vi "Ref AVI Video-Generate file name.vi"(8 "error in (no error)":errorcluster, 9 "Channel":T1, 11 "Videos folder path":path) -> (0 "error out":errorcluster, 3 "AVI file path & name":path)   [LabVIEW 2020]
uses:
  Typedefs/Channel Selector.ctl
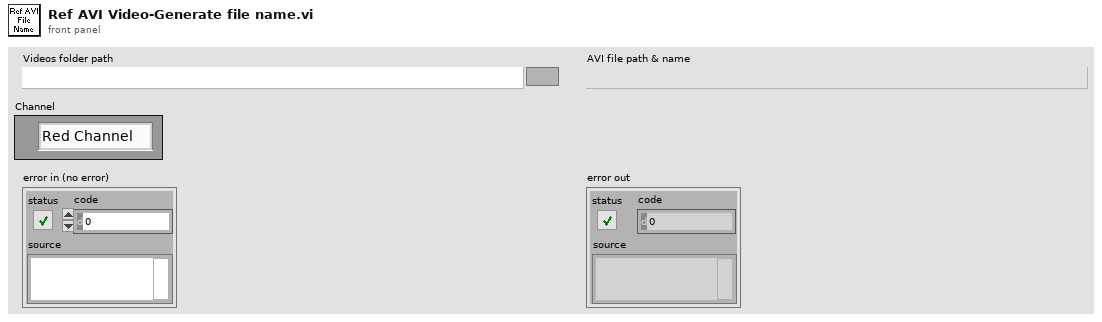
[diagram p1: front panel]
types:
  T1 = typedef "Channel Selector.ctl" = enum16{"Red Channel", "Green Channel", "Blended"}
  T2 = typedef "AVI Refs cluster.ctl" = cluster{"AVI2 path":path, "AVI 2 Refnum":T3, "New Image":T4, "error out":errorcluster, "Avi 1 Refnum":T5}
  T3 = typedef "IMAQ AVI2 Refnum.ctl" = refnum<k20>
  T4 = typedef "IMAQ Image.ctl" = refnum<image>
  T5 = typedef "AviRefnum.ctl" = refnum<k1>
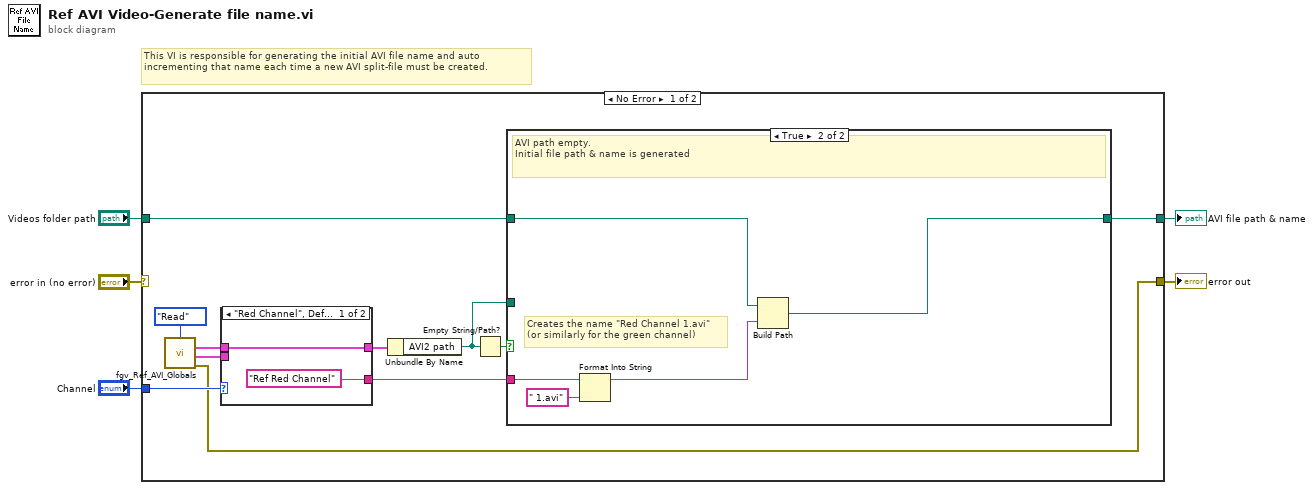
[diagram p0: block diagram]
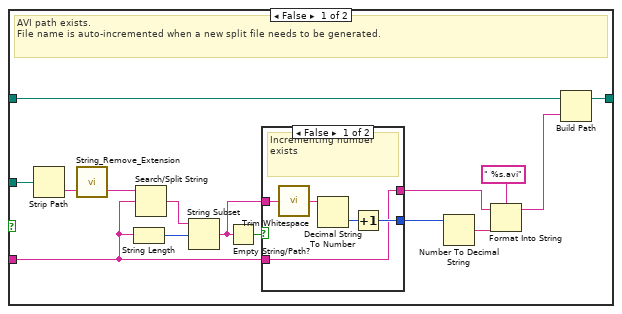
[diagram p2: hidden frame]
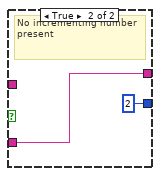
[diagram p3: hidden frame]
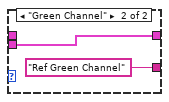
[diagram p4: hidden frame]
diagram:
  # "This VI is responsible for generating the initial AVI file name and auto incrementing that name each time a new AVI split-file must be created."
  n1 = case shown="No Error" "error in (no error)" {
    selector: "error in (no error)" -> [_ w49]
    tunnel: "Videos folder path" -> [w11 w48]
    tunnel: [w9 w48] -> w4
    tunnel: [w7 w49] -> w3
    tunnel: "Channel" -> [w8 _]
    frame No Error {
      n2 = call "fgv_Ref_AVI_Globals.vi"("Function"=enum16{"Intialize", "Write", "Read", "Clear"}."Read") -> ("Red Ref AVI"=w14:T2, "Green Ref AVI"=w15:T2, "error out"=w7:errorcluster)  [unwired: 11 in, 1 out]
      n3 = case shown="\"Red Channel\", Default" w8 {
        tunnel: w14 -> [w45 _]
        tunnel: w15 -> [_ w47]
        tunnel: [w45 w47] -> w16
        tunnel: ["Ref Red Channel" ("name or relative path") "Ref Green Channel" ("name or relative path")] -> w6
        frame "Red Channel", Default {
        }
        frame "Green Channel" {
        }
      }
      n4 = Unbundle By Name(w16) -> ("AVI2 path"=w10:path)
      n5 = Empty String/Path?(string/path=w10) -> (empty?=w12:bool)
      n6 = case shown="True" w12 {
        tunnel: w11 -> [w23 w43]
        tunnel: [w31 w42] -> w9
        tunnel: w10 -> [w22 _]
        tunnel: w6 -> [w17 w41]
        frame False {
          # "AVI path exists.\nFile name is auto-incremented when a new split file needs to be generated."
          n7 = Strip Path(path=w22) -> (name=w30:string)  [unwired: 1 out]
          n8 = call <userlib>:"String_Remove_Extension.vi"("File name with extension"=w30) -> ("Filename without extension"=w21:string)  [unwired: 1 in, 1 out]
          n9 = String Length(string=w17) -> (length=w19:i32)
          n10 = Search/Split String(string=w21, search string/char (-)=w17) -> (match + rest of string=w20:string)  [unwired: 1 in, 2 out]
          n11 = String Subset(string=w20, offset (0)=w19) -> (substring=w18:string)  [unwired: 1 in]
          n12 = Empty String/Path?(string/path=w18) -> (empty?=w29:bool)
          n13 = case shown="False" w29 {
            tunnel: w18 -> [w35 _]
            tunnel: [w33 2] -> w25
            tunnel: [w32 w37] -> w24
            tunnel: w17 -> [w32 w37]
            frame False {
              # "Incrementing number exists"
              n14 = call <vilib>:"Trim Whitespace.vi"("string"=w35) -> ("trimmed string"=w36:string)  [unwired: 1 in]
              n15 = Decimal String To Number(string=w36) -> (number=w34:i32)  [unwired: 2 in, 1 out]
              n16 = Increment(x=w34) -> (x+1=w33:i32)
            }
            frame True {
              # "No incrementing number present"
            }
          }
          n17 = Number To Decimal String(number=w25) -> (decimal integer string=w28:string)  [unwired: 1 in]
          n18 = Format Into String(format string=" %s.avi", initial string=w24, w28) -> (resulting string=w26:string)  [unwired: 1 in, 1 out]
          n19 = Build Path(base path=w23, name or relative path=w26) -> (appended path=w31:path)
        }
        frame True {
          # "Creates the name \"Red Channel 1.avi\"\n(or similarly for the green channel)"
          # "AVI path empty.\nInitial file path & name is generated"
          n20 = Format Into String(initial string=w41, " 1.avi" ("format string")) -> (resulting string=w39:string)  [unwired: 2 in, 1 out]
          n21 = Build Path(base path=w43, name or relative path=w39) -> (appended path=w42:path)
        }
      }
    }
    frame Error {
    }
  }
  "AVI file path & name" <- w4
  "error out" <- w3
